vi "BACKTOBASE2.vi"   [LabVIEW 2016, in "Test2.lvrbt"]
uses:
  Test2.lvrbt
  <vilib>/NXT/Subs/ColorSensorColors.ctl
  <vilib>/NXT/Block Support/NXT_InputPort.ctl
  <vilib>/NXT/Hardware/Plugins/Tetrix DC Motor/TetrixDCMotorAddress.ctl
  <vilib>/NXT/Hardware/Plugins/Tetrix 180 deg Servo/Tetrix180ServoAddress.ctl
  <vilib>/NXT/NXTIO Xnodes/NXTIONodeSubVIs/TETRIX IO Move DC Motors.vi
  <vilib>/NXT/Dual Mode Library/Waits/Wait_Num.vi
  <vilib>/NXT/NXTIO Xnodes/NXTIONodeSubVIs/TETRIX IO Stop DC Motors.vi
  <vilib>/NXT/Dual Mode Library/Waits/Wait_EV3_Color_Color.vi
  <vilib>/NXT/NXTIO Xnodes/NXTIONodeSubVIs/TETRIX IO Move Servos.vi
  <vilib>/NXT/Subs/LVHSConnector.ctl
  <vilib>/NXT/NXTIO Xnodes/AddressXNode/NXTIOAddress.xnode
  <vilib>/NXT/NXTIO Xnodes/NXTIOXNode/NXTIO.xnode
  <vilib>/NXT/LegoClasses/BrickReference/BrickReference.lvclass
types:
  T1 = typedef "NXT_InputPort.ctl" = u32
  T2 = typedef "ColorSensorColors.ctl" = enum16{"No Color", "Black", "Blue", "Green", "Yellow", "Red", "White", "Brown"}
  T3 = typedef "TetrixDCMotorAddress.ctl" = i32
  T4 = typedef "LVHSConnector.ctl" = refnum<class "BrickReference.lvclass">
  T5 = typedef "Tetrix180ServoAddress.ctl" = i32
  T6 = cluster{"Tetrix180Servo":T5, "Tetrix180Servo":T5, "Tetrix180Servo":T5, "Tetrix180Servo":T5, "Tetrix180Servo":T5, "Tetrix180Servo":T5}
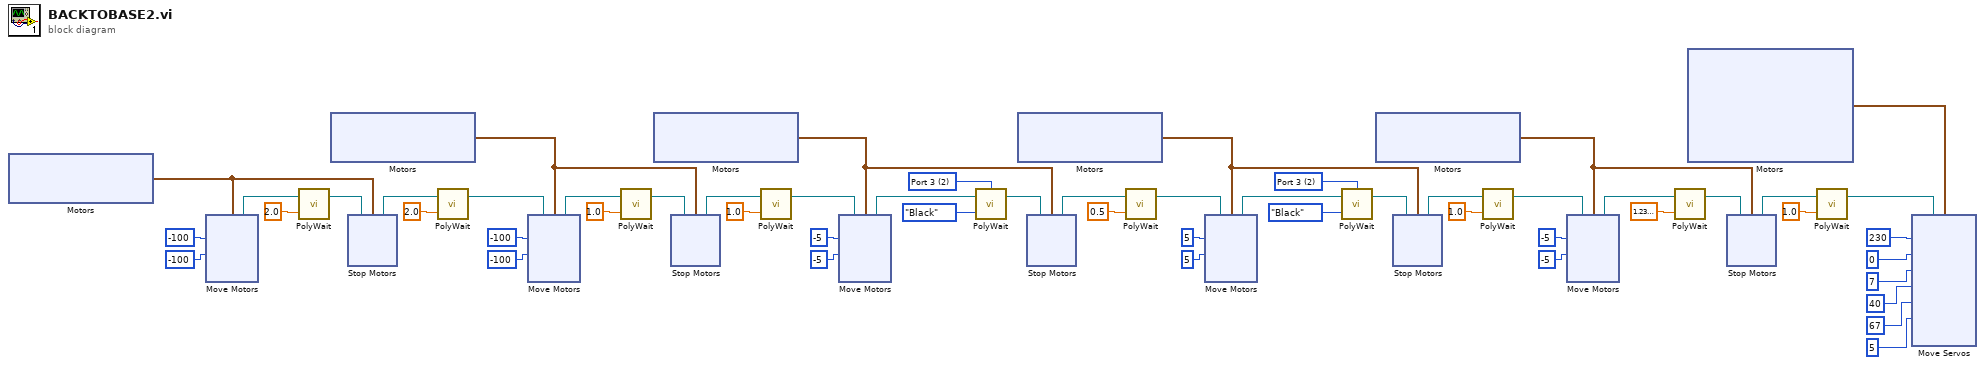
[diagram p0: block diagram]
diagram:
  w2 = T1 2 items=["Port 1", "Port 2", "Port 3", "Port 4"] ("Port (Port 1)")
  w30 = T1 2 items=["Port 1", "Port 2", "Port 3", "Port 4"] ("Port (Port 1)")
  n1 = xnode "Motors"() -> ("Motor"=w49:cluster{"TetrixDCMotor":T3, "TetrixDCMotor":T3})
  n2 = xnode "Move Motors"("Power/Speed 2"=i8 -100, "Power/Speed 1"=i8 -100, "Motors"=w49) -> ("NXT/EV3"=w52:T4)  [unwired: 1 in]
  n3 = call-poly <vilib>:"PolyWait.vi"("Time (1 sec)"=sgl 2.0, "NXT/EV3"=w52) -> ("NXT/EV3"=w50:T4)  [unwired: 2 in]
  n4 = xnode "Motors"() -> ("Motor"=w43:cluster{"TetrixDCMotor":T3, "TetrixDCMotor":T3})
  n5 = xnode "Stop Motors"("Motors"=w49, "NXT/EV3"=w50) -> ("NXT/EV3"=w41:T4)
  n6 = call-poly <vilib>:"PolyWait.vi"("Time (1 sec)"=sgl 2.0, "NXT/EV3"=w41) -> ("NXT/EV3"=w40:T4)  [unwired: 2 in]
  n7 = xnode "Move Motors"("Power/Speed 2"=i8 -100, "Power/Speed 1"=i8 -100, "Motors"=w43, "NXT/EV3"=w40) -> ("NXT/EV3"=w46:T4)
  n8 = call-poly <vilib>:"PolyWait.vi"("Time (1 sec)"=sgl 1.0, "NXT/EV3"=w46) -> ("NXT/EV3"=w44:T4)  [unwired: 2 in]
  n9 = xnode "Motors"() -> ("Motor"=w33:cluster{"TetrixDCMotor":T3, "TetrixDCMotor":T3})
  n10 = xnode "Stop Motors"("Motors"=w43, "NXT/EV3"=w44) -> ("NXT/EV3"=w38:T4)
  n11 = call-poly <vilib>:"PolyWait.vi"("Time (1 sec)"=sgl 1.0, "NXT/EV3"=w38) -> ("NXT/EV3"=w32:T4)  [unwired: 2 in]
  n12 = xnode "Move Motors"("Power/Speed 2"=i8 -5, "Power/Speed 1"=i8 -5, "Motors"=w33, "NXT/EV3"=w32) -> ("NXT/EV3"=w35:T4)
  n13 = call-poly <vilib>:"PolyWait.vi"("Color (Red)"=ColorSensorColors."Black", "NXT/EV3"=w35, "Port (Port 1)"=w30) -> ("NXT/EV3"=w34:T4)  [unwired: 1 in]
  n14 = xnode "Motors"() -> ("Motor"=w24:cluster{"TetrixDCMotor":T3, "TetrixDCMotor":T3})
  n15 = xnode "Stop Motors"("Motors"=w33, "NXT/EV3"=w34) -> ("NXT/EV3"=w3:T4)
  n16 = call-poly <vilib>:"PolyWait.vi"("Time (1 sec)"=sgl 0.5, "NXT/EV3"=w3) -> ("NXT/EV3"=w13:T4)  [unwired: 2 in]
  n17 = xnode "Move Motors"("Power/Speed 2"=i8 5, "Power/Speed 1"=i8 5, "Motors"=w24, "NXT/EV3"=w13) -> ("NXT/EV3"=w25:T4)
  n18 = call-poly <vilib>:"PolyWait.vi"("Color (Red)"=ColorSensorColors."Black", "NXT/EV3"=w25, "Port (Port 1)"=w2) -> ("NXT/EV3"=w26:T4)  [unwired: 1 in]
  n19 = xnode "Motors"() -> ("Motor"=w15:cluster{"TetrixDCMotor":T3, "TetrixDCMotor":T3})
  n20 = xnode "Stop Motors"("Motors"=w24, "NXT/EV3"=w26) -> ("NXT/EV3"=w22:T4)
  n21 = call-poly <vilib>:"PolyWait.vi"("Time (1 sec)"=sgl 1.0, "NXT/EV3"=w22) -> ("NXT/EV3"=w19:T4)  [unwired: 2 in]
  n22 = xnode "Move Motors"("Power/Speed 2"=i8 -5, "Power/Speed 1"=i8 -5, "Motors"=w15, "NXT/EV3"=w19) -> ("NXT/EV3"=w17:T4)
  n23 = call-poly <vilib>:"PolyWait.vi"("Time (1 sec)"=sgl 1.23, "NXT/EV3"=w17) -> ("NXT/EV3"=w16:T4)  [unwired: 2 in]
  n24 = xnode "Motors"() -> ("Motor"=w10:T6)
  n25 = xnode "Stop Motors"("Motors"=w15, "NXT/EV3"=w16) -> ("NXT/EV3"=w12:T4)
  n26 = call-poly <vilib>:"PolyWait.vi"("Time (1 sec)"=sgl 1.0, "NXT/EV3"=w12) -> ("NXT/EV3"=w4:T4)  [unwired: 2 in]
  n27 = xnode "Move Servos"("Position 6"=u8 5, "Position 5"=u8 67, "Position 4"=u8 40, "Position 3"=u8 7, "Position 2"=u8 0, "Position 1"=u8 230, "Motors"=w10, "NXT/EV3"=w4) -> ()  [unwired: 1 out]
